vi "Read Multiple.vi"(0 "RS232 Port In":refnum<visa-resource-name>, 1 "Sensor Address In Array":string[](array[string]), 4 "Measurement Type In (Normal)":i32(ring) items=["Normal", "Concurrent", "Continuous"], 5 "CRC In Array (False)":bool[](array[boolean]), 6 "Parameter In Array (0)":i32[](array[ring]) items=["0", "1", "2", "3", "4", "5", "6", "7", "8", "9"], 7 "Error In (No Error)":errorcluster) -> (20 "RS232 Port Out":refnum<visa-resource-name>="COM1", 21 "Sensor Address Out Array":string[](array[string]), 22 "Measurements Out":dbl[][](array[numeric]), 23 "Number of Measurements Out Array":i32[](array[numeric]), 24 "Measurement Type Out":i32(ring) items=["Normal", "Concurrent", "Continuous"], 25 "CRC Out Array":bool[](array[boolean]), 26 "Parameter Out Array":i32[](array[ring]) items=["0", "1", "2", "3", "4", "5", "6", "7", "8", "9"], 27 "Error Out Array":errorcluster[](array[cluster]))   [LabVIEW 2016, in "SDI-12.lvlib"]
doc: "Creates and sends multiple measurement commands to sensor(s), and reads the measurement responses. Provide this VI with an array of sensor addresses, the measurement type (scalar for all measurements), an array of signal parameters, and an array of CRC booleans. \n\nEach array's index correlate into settings for a single measurement, which may return between 1 and 20 data points as specified in the SDI-12 protocol version 1.3. The amount of data measured depends on settings of each sensor, and these settings are not ecompassed by the SDI-12 protocol.\n\nVisit http://www.sdi-12.org/ for more information on the SDI-12 protocol."
uses:
  SDI-12.lvlib
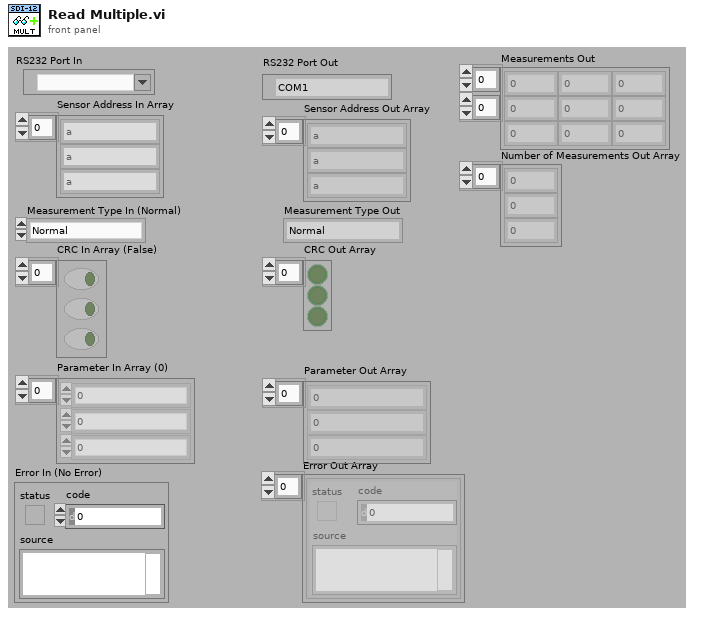
[diagram p1: front panel]
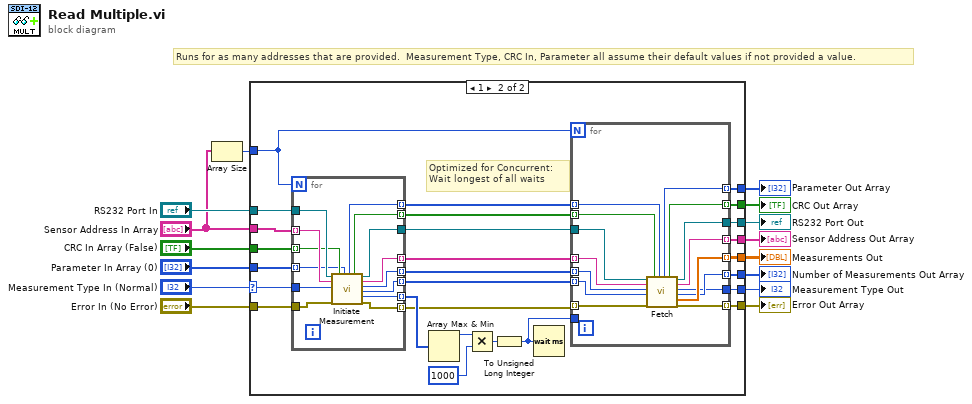
[diagram p0: block diagram]
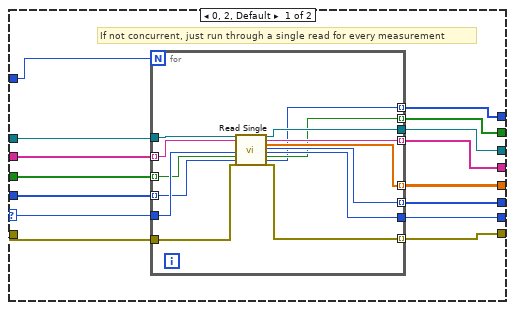
[diagram p2: hidden frame]
diagram:
  # "Runs for as many addresses that are provided.  Measurement Type, CRC In, Parameter all assume their default values if not provided a value."
  n1 = Array Size(array="Sensor Address In Array") -> (size(s)=w12:i32)
  n2 = case shown="1" "Measurement Type In (Normal)" {
    selector: "Measurement Type In (Normal)" -> [w24 w47]
    tunnel: "RS232 Port In" -> [w29 w71]
    tunnel: "Error In (No Error)" -> [w25 w70]
    tunnel: "CRC In Array (False)" -> [w27 w69]
    tunnel: "Parameter In Array (0)" -> [w26 w68]
    tunnel: w12 -> [w30 w46]
    tunnel: "Sensor Address In Array" -> [w28 w67]
    tunnel: [w23 w54] -> w9
    tunnel: [w20 w45] -> w8
    tunnel: [w19 w53] -> w7
    tunnel: [w21 w52] -> w6
    tunnel: [w18 w51] -> w5
    tunnel: [w22 w50] -> w4
    tunnel: [w17 w49] -> w3
    tunnel: [w16 w48] -> w2
    frame 0, 2, Default {
      # "If not concurrent, just run through a single read for every measurement"
      n3 = for {
        N: w30 -> [_]
        tunnel: w29 -> [w44]
        tunnel: w25 -> [w40]
        tunnel: w28 -> [w31] mode=indexing
        tunnel: w27 -> [w42] mode=indexing
        tunnel: w26 -> [w41] mode=indexing
        tunnel: w24 -> [w43]
        tunnel: [w39] -> w23 mode=indexing
        tunnel: [w38] -> w22
        tunnel: [w37] -> w21 mode=indexing
        tunnel: [w36] -> w20 mode=indexing
        tunnel: [w35] -> w19 mode=indexing
        tunnel: [w34] -> w18
        tunnel: [w33] -> w17 mode=indexing
        tunnel: [w32] -> w16 mode=indexing
        n4 = call "Read Single.vi"("RS232 Port In"=w44, "Sensor Address In"=w31, "Measurement Type In (Normal)"=w43, "CRC (False)"=w42, "Parameter In (0)"=w41, "Error In (No Error)"=w40) -> ("RS232 Port Out"=w38:refnum<visa-resource-name>, "Sensor Address Out"=w37:string, "Measurements Out"=w36:dbl[], "Number of Measurements Out"=w35:i32, "Measurement Type Out"=w34:i32, "CRC Out"=w33:bool, "Parameter Out"=w32:i32, "Error Out"=w39:errorcluster)  [unwired: 14 in]
      }
    }
    frame 1 {
      # "Optimized for Concurrent:\nWait longest of all waits"
      n5 = for {
        N: w46 -> [_]
        tunnel: w71 -> [w100]
        tunnel: w70 -> [w97]
        tunnel: w67 -> [w99] mode=indexing
        tunnel: w69 -> [w98] mode=indexing
        tunnel: w68 -> [w96] mode=indexing
        tunnel: [w92] -> w58
        tunnel: [w95] -> w57 mode=indexing
        tunnel: [w94] -> w60 mode=indexing
        tunnel: [w93] -> w59 mode=indexing
        tunnel: [w91] -> w56 mode=indexing
        tunnel: [w90] -> w55 mode=indexing
        tunnel: w47 -> [w89]
        tunnel: [w88] -> w66 mode=indexing
        tunnel: [w87] -> w61 mode=indexing
        n6 = call "Initiate Measurement.vi"("RS232 Port In"=w100, "Sensor Address In"=w99, "Measurement Type In (Normal)"=w89, "Error In (No Error)"=w97, "CRC In (False)"=w98, "Parameter In (0)"=w96) -> ("Parameter Out"=w94:i32, "CRC Out"=w93:bool, "RS232 Port Out"=w92:refnum<visa-resource-name>, "Sensor Address Out"=w95:string, "Measurement Type Out"=w91:i32, "Number of Measurements"=w90:i32, "Max Acquisition Time (sec)"=w88:i32, "Error Out"=w87:errorcluster)  [unwired: 6 in]
      }
      n7 = Array Max & Min(array=w66) -> (max value=w65:i32)  [unwired: 3 out]
      n8 = Multiply(x=w65, y=1000) -> (x*y=w63:i32)
      n9 = To Unsigned Long Integer(number=w63) -> (unsigned 32bit integer=w62:u32)
      n10 = Wait (ms)(milliseconds to wait=w62) -> ()  [unwired: 1 out]
      n11 = for {
        N: w46 -> [_]
        tunnel: w61 -> [w86] mode=indexing
        tunnel: w62 -> [_]
        tunnel: w60 -> [w80] mode=indexing
        tunnel: w59 -> [w81] mode=indexing
        tunnel: w58 -> [w82]
        tunnel: w57 -> [w83] mode=indexing
        tunnel: w56 -> [w84] mode=indexing
        tunnel: w55 -> [w85] mode=indexing
        tunnel: [w79] -> w54 mode=indexing
        tunnel: [w78] -> w45 mode=indexing
        tunnel: [w77] -> w53 mode=indexing
        tunnel: [w76] -> w52 mode=indexing
        tunnel: [w75] -> w51
        tunnel: [w74] -> w50
        tunnel: [w73] -> w49 mode=indexing
        tunnel: [w72] -> w48 mode=indexing
        n12 = call "Fetch.vi"("RS232 Port In"=w82, "Sensor Address In"=w83, "Measurement Type In (Normal)"=w84, "Number of Measurements In (1)"=w85, "Error In (No Error)"=w86, "CRC (False)"=w81, "Parameter In (0)"=w80) -> ("Parameter Out"=w72:i32, "CRC Out"=w73:bool, "RS232 Port Out"=w74:refnum<visa-resource-name>, "Sensor Address Out"=w76:string, "Measurement Type Out"=w75:i32, "Number of Measurements Out"=w77:i32, "Measurements Out"=w78:dbl[], "Error Out"=w79:errorcluster)  [unwired: 5 in]
      }
    }
  }
  "Measurements Out" <- w8
  "Error Out Array" <- w9
  "CRC Out Array" <- w3
  "Sensor Address Out Array" <- w6
  "Parameter Out Array" <- w2
  "Number of Measurements Out Array" <- w7
  "RS232 Port Out" <- w4
  "Measurement Type Out" <- w5
